vi "Tempeature Warnings.vi"(8 "error in (no error)":errorcluster, 11 "Weather Data In":T1={"Current Temperature"=0.0, "Max Temperature"=0.0, "Min Temperature"=0.0, "Warning Text"="", "Warning?"=FALSE, "Enum"=enum."Fahrenheit", "Current Windspeed"=0.0, "Max Windspeed"=0.0, "Windspeed Warning?"=FALSE, "Windspeed Warning Text"="No Warning"}) -> (0 "error out":errorcluster, 3 "Weather Data out":T1={"Current Temperature"=0.0, "Max Temperature"=0.0, "Min Temperature"=0.0, "Warning Text"="", "Warning?"=FALSE, "Enum"=enum."Fahrenheit", "Current Windspeed"=0.0, "Max Windspeed"=0.0, "Windspeed Warning?"=FALSE, "Windspeed Warning Text"="No Warning"})   [LabVIEW 2012]
doc: "Weather warning VI. Outputs warning based on current temperature in comparison with min or max temperature\n\nJaskaran Dhiman\n6/24/2013"
uses:
  weather data.ctl
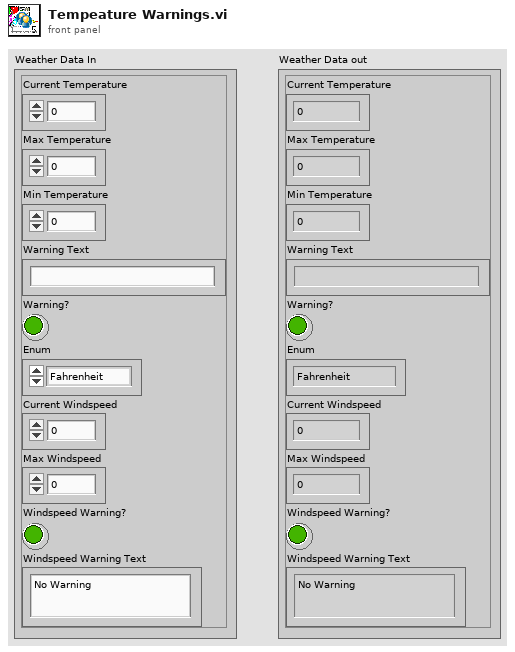
[diagram p1: front panel]
types:
  T1 = typedef "weather data.ctl" = cluster{"Current Temperature":dbl, "Max Temperature":dbl, "Min Temperature":dbl, "Warning Text":string, "Warning?":bool, "Enum":enum16{"Fahrenheit", "Celcius"}, "Current Windspeed":dbl, "Max Windspeed":dbl, "Windspeed Warning?":bool, "Windspeed Warning Text":string}
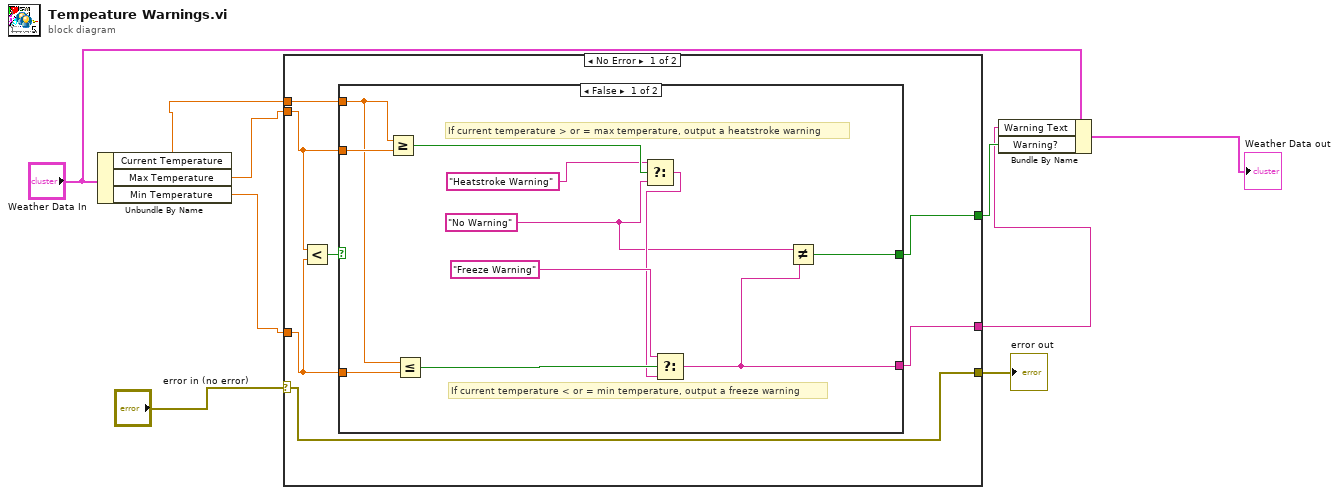
[diagram p0: block diagram]
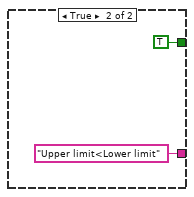
[diagram p2: hidden frame]
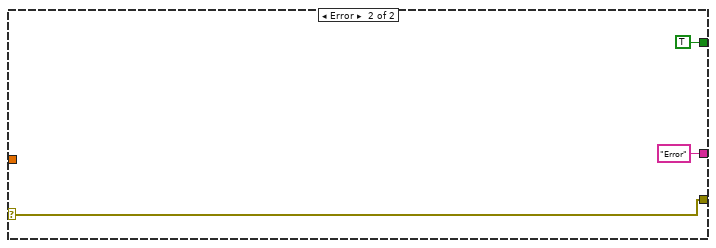
[diagram p3: hidden frame]
diagram:
  n1 = Unbundle By Name("Weather Data In") -> ("Current Temperature"=w7:dbl, "Max Temperature"=w6:dbl, "Min Temperature"=w5:dbl)
  n2 = case shown="No Error" "error in (no error)" {
    selector: "error in (no error)" -> [w14 w31]
    tunnel: w5 -> [w10 _]
    tunnel: w7 -> [w13 _]
    tunnel: [w16 "Error"] -> w1
    tunnel: [w15 TRUE] -> w2
    tunnel: w6 -> [w11 _]
    tunnel: [w14 w31] -> w8
    frame No Error {
      n3 = Less?(x=w11, y=w10) -> (x < y?=w12:bool)
      n4 = case shown="False" w12 {
        tunnel: [w21 "Upper limit<Lower limit"] -> w16
        tunnel: [w20 TRUE] -> w15
        tunnel: w13 -> [w17 _]
        tunnel: w11 -> [w19 _]
        tunnel: w10 -> [w18 _]
        frame False {
          w22 = "No Warning"
          # "If current temperature < or = min temperature, output a freeze warning"
          # "If current temperature > or = max temperature, output a heatstroke warning"
          n5 = Greater Or Equal?(x=w17, y=w19) -> (x >= y?=w27:bool)
          n6 = Less Or Equal?(x=w17, y=w18) -> (x <= y?=w25:bool)
          n7 = Select(t="Heatstroke Warning", s=w27, f=w22) -> (s? t:f=w23:string)
          n8 = Select(t="Freeze Warning", s=w25, f=w23) -> (s? t:f=w21:string)
          n9 = Not Equal?(x=w22, y=w21) -> (x != y?=w20:bool)
        }
        frame True {
        }
      }
    }
    frame Error {
    }
  }
  "error out" <- w8
  n10 = Bundle By Name(cluster="Weather Data In", "Warning Text"=w1, "Warning?"=w2) -> (→"Weather Data out":T1)
